vi "HTR_Test.vi"(0 "CurrentTest":T2 {"Post-Log(s)" format="%#_13g"; "Pre-Log (s)" format="%#_13g"; "Duration (s)" format="%#_13g"}, 1 "Status Ref":refnum<vi>, 2 "HTR_Monitor Ref":refnum<vi>, 3 "HTR_OnOff Ref":refnum<vi>, 5 "Heater Test Options":T1 {"Heater Voltage Tolerance (%)" min=1.0 max=100.0; "Heater Nominal Voltage (V)" min=0.0 max=1.0}, 9 "HTR Fault Ref":refnum<vi>, 11 "error in (no error)":errorcluster, 12 "DelayRemaining":refnum<vi>, 14 "HTR_Enable Ref":refnum<vi>) -> (15 "error out":errorcluster)   [LabVIEW 2025]
uses:
  controls/SingleTest.ctl
  controls/TestType.ctl
  controls/HTR Test Options.ctl
  <userlib>/_OpenG.lib/time/time.llb/openg_time.lvlib
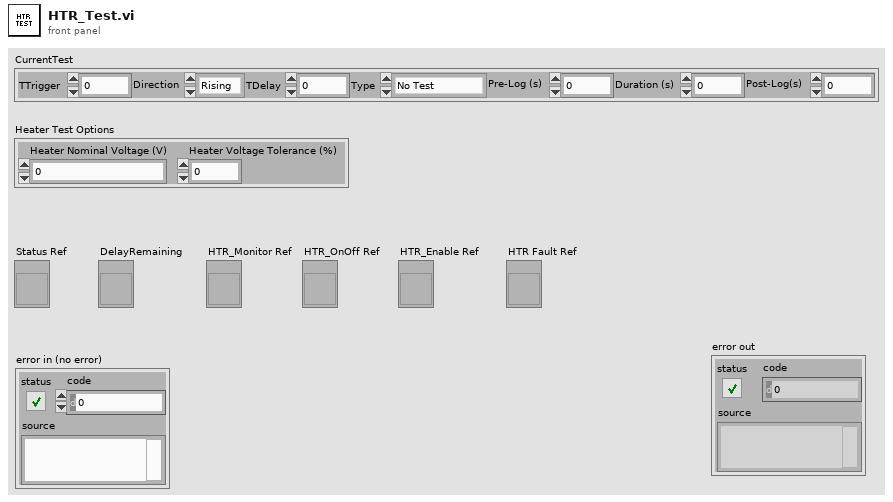
[diagram p1: front panel]
types:
  T1 = typedef "HTR Test Options.ctl" = cluster{"Heater Nominal Voltage (V)":dbl, "Heater Voltage Tolerance (%)":dbl}
  T2 = typedef "SingleTest.ctl" = cluster{"TTrigger":dbl, "Direction":enum16{"Rising", "Falling"}, "TDelay":dbl, "Type":T3, "Pre-Log (s)":dbl, "Duration (s)":dbl, "Post-Log(s)":dbl}
  T3 = typedef "TestType.ctl" = enum16{"No Test", "Heater Test", "Actuation Test", "Diode Test"}
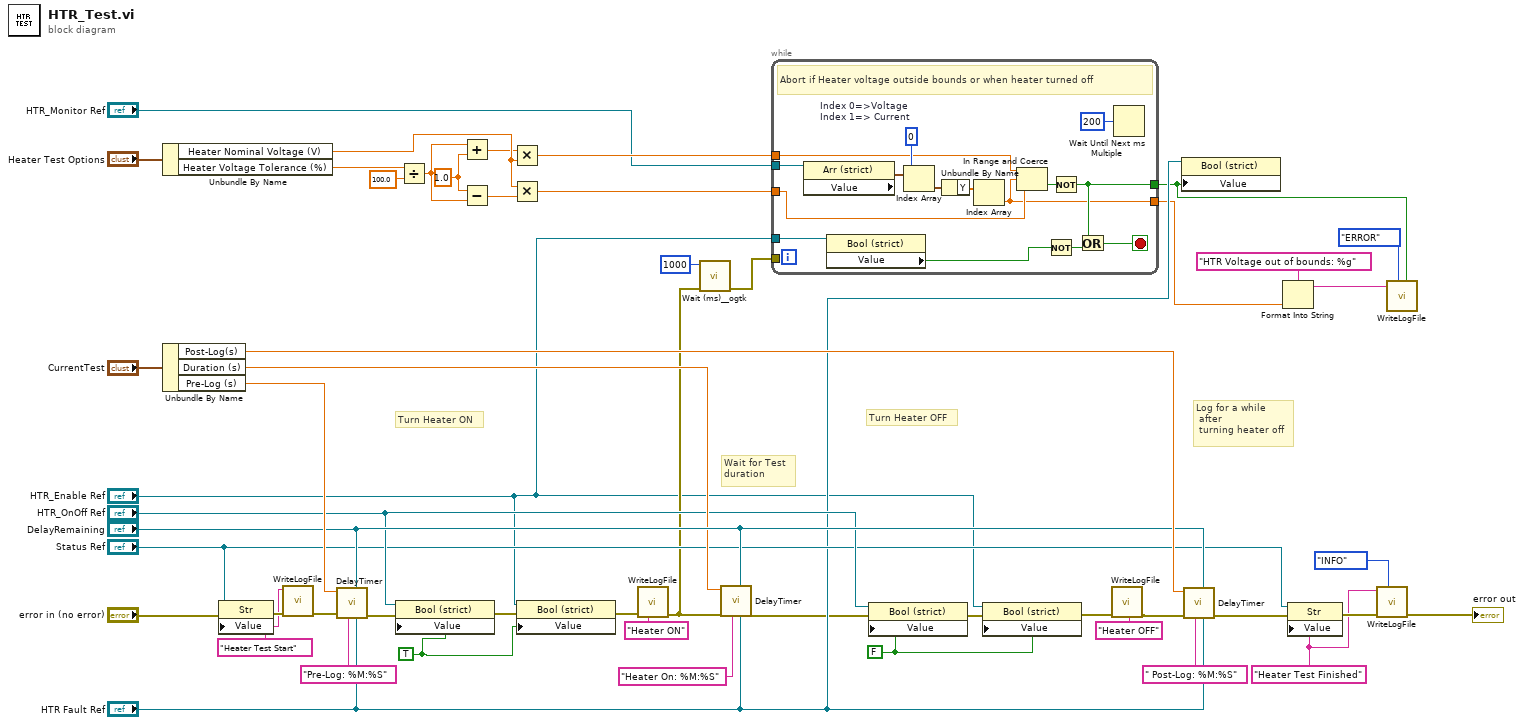
[diagram p0: block diagram]
diagram:
  w30 = 1.0 ("x")
  w4 = "Heater Test Finished" ("Status")
  w38 = TRUE ("Heater Logging")
  w46 = FALSE ("Heater PSU")
  w24 = "Heater Test Start" ("Status")
  # "Log for a while\n after\n turning heater off"
  # "Wait for Test \nduration"
  # "Turn Heater OFF"
  # "Turn Heater ON"
  n1 = Unbundle By Name("Heater Test Options") -> ("Heater Nominal Voltage (V)"=w34:dbl, "Heater Voltage Tolerance (%)"=w28:dbl)
  n2 = Unbundle By Name("CurrentTest") -> ("Post-Log(s)"=w50:dbl, "Duration (s)"=w42:dbl, "Pre-Log (s)"=w51:dbl)
  n3 = property on="Property Node" class="Str"(reference="Status Ref", error in="error in (no error)", "Value"=w24) -> (error out=w25:errorcluster)  [unwired: 1 out]
  n4 = call "WriteLogFile.vi"("error in (no error)"=w25, "Message"=w24) -> ("error out"=w26:errorcluster)  [unwired: 9 in]
  n5 = call "DelayTimer.vi"("Abort Ref"="HTR Fault Ref", "Formatted \nTime Ref"="DelayRemaining", "FormatString"="Pre-Log: %M:%S", "error in (no error)"=w26, "Delay(s)"=w51) -> ("error out"=w43:errorcluster)  [unwired: 6 in]
  n6 = property on="Property Node" class="Bool (strict)"(reference="HTR_OnOff Ref", error in=w43, "Value"=w38) -> (error out=w39:errorcluster)  [unwired: 1 out]
  n7 = Divide(x=w28, y=100.0) -> (x/y=w31:dbl)
  n8 = Add(x=w31, y=w30) -> (x+y=w32:dbl)
  n9 = Subtract(x=w30, y=w31) -> (x-y=w33:dbl)
  n10 = Multiply(x=w32, y=w34) -> (x*y=w21:dbl)
  n11 = Multiply(x=w34, y=w33) -> (x*y=w20:dbl)
  n12 = property class="Bool (strict)"(reference="HTR_Enable Ref", error in=w39, "Value"=w38) -> (error out=w23:errorcluster)  [unwired: 1 out]
  n13 = call "WriteLogFile.vi"("error in (no error)"=w23, "Message"="Heater ON") -> ("error out"=w18:errorcluster)  [unwired: 9 in]
  n14 = call <userlib>:"Wait (ms)__ogtk.vi"("error in (no error)"=w18, "milliseconds to wait"=u32 1000) -> ("error out"=w3:errorcluster)  [unwired: 8 in, 1 out]
  n15 = call "DelayTimer.vi"("Abort Ref"="HTR Fault Ref", "Formatted \nTime Ref"="DelayRemaining", "FormatString"="Heater On: %M:%S", "error in (no error)"=w18, "Delay(s)"=w42) -> ("error out"=w8:errorcluster)  [unwired: 6 in]
  n16 = while {
    tunnel: w21 -> [w62]
    tunnel: w20 -> [w61]
    tunnel: [w58] -> w11
    tunnel: "HTR_Monitor Ref" -> [w55]
    tunnel: "HTR_Enable Ref" -> [w54]
    tunnel: w3 -> [_]
    tunnel: [w52] -> w14
    stop <- w57 stop-if-true
    w65 = 0  # Index 0=>Voltage Index 1=> Current
    # "Abort if Heater voltage outside bounds or when heater turned off"
    n17 = property class="Arr (strict)"(reference=w55) -> ("Value"=w66:waveform(dbl)[])  [unwired: 1 in, 2 out]
    n18 = property class="Bool (strict)"(reference=w54) -> ("Value"=w59:bool)  [unwired: 1 in, 2 out]
    n19 = Index Array(array=w66, index=w65) -> (element=w64:waveform(dbl))
    n20 = Unbundle By Name(w64) -> ("Y"=w63:dbl[])
    n21 = Index Array(array=w63) -> (element=w52:dbl)  [unwired: 1 in]
    n22 = In Range and Coerce(upper limit=w62, x=w52, lower limit=w61) -> (In Range?=w60:bool)  [unwired: 1 out]
    n23 = Not(x=w59) -> (.not. x?=w56:bool)
    n24 = Not(x=w60) -> (.not. x?=w58:bool)
    n25 = Or(x=w58, y=w56) -> (x .or. y?=w57:bool)
    n26 = Wait Until Next ms Multiple(millisecond multiple=u32 200) -> ()  [unwired: 1 out]
  }
  n27 = property on="Property Node" class="Bool (strict)"(reference="HTR_OnOff Ref", error in=w8, "Value"=w46) -> (error out=w40:errorcluster)  [unwired: 1 out]
  n28 = property class="Bool (strict)"(reference="HTR_Enable Ref", error in=w40, "Value"=w46) -> (error out=w9:errorcluster)  [unwired: 1 out]
  n29 = call "WriteLogFile.vi"("error in (no error)"=w9, "Message"="Heater OFF") -> ("error out"=w10:errorcluster)  [unwired: 9 in]
  n30 = property class="Bool (strict)"(reference="HTR Fault Ref", "Value"=w11) -> ()  [unwired: 1 in, 2 out]
  n31 = call "DelayTimer.vi"("Abort Ref"="HTR Fault Ref", "Formatted \nTime Ref"="DelayRemaining", "FormatString"=" Post-Log: %M:%S", "error in (no error)"=w10, "Delay(s)"=w50) -> ("error out"=w37:errorcluster)  [unwired: 6 in]
  n32 = Format Into String(format string="HTR Voltage out of bounds: %g", w14) -> (resulting string=w13:string)  [unwired: 2 in, 1 out]
  n33 = property on="Property Node" class="Str"(reference="Status Ref", error in=w37, "Value"=w4) -> (error out=w7:errorcluster)  [unwired: 1 out]
  n34 = call "WriteLogFile.vi"("Type"=enum16{"INFO", "WARNING", "ERROR"}."INFO", "error in (no error)"=w7, "Message"=w4) -> ("error out"=→"error out":errorcluster)  [unwired: 8 in]
  n35 = call "WriteLogFile.vi"("Write?"=w11, "Type"=enum16{"INFO", "WARNING", "ERROR"}."ERROR", "Message"=w13) -> ()  [unwired: 8 in, 1 out]
